vi "Example - DataType Datatype Check.vi"() -> ()   [LabVIEW 2017]
uses:
  API-String-Arugments-Support/API String Arguments Support.lvlib
panel:
  in  "String 32":string=" -4.86725 "
  out "error 16":errorcluster
  out "Data 15":cdb=-4.86725+0.0i
  out "String 31":string="-4.86725 +0i"
  in  "String 30":string="-3.14i "
  out "error 15":errorcluster
  out "Data 14":cdb=-3.14+0.0i
  out "String 29":string="-3.14 +0i"
  in  "String 28":string=" -4.86725 +3.14i "
  out "error 14":errorcluster
  out "Data 13":cdb=-4.86725+3.14i
  out "String 27":string="-4.86725 +3.14i"
  in  "String 26":string=" 4.86725 +3.14i "
  out "error 13":errorcluster
  out "Data 12":cdb=4.86725+3.14i
  out "String 25":string="4.86725 +3.14i"
  out "String 24":string="abcd"
  out "String 23":string="TRUE"
  out "String 22":string="66"
  out "String 21":string="3.1415926"
  out "String 20":string="bbbb"
  out "String 19":string="555 - ccccc"
  out "String 18":string="555 - ccccc"
  out "String 17":string="[3.12,4.11,5]"
  out "String 16":string="{Name:abc;Child.Name:ddd;Bool:FALSE}"
  out "String 15":string="C:\\ni-rt\\data\\a\\2023.07.25"
  out "String 14":string="[{Name:;Child.Name:ddd;Bool:FALSE},{Name:ddd;Child.Name:;Bool:TRUE}]"
  out "String 13":string="[3.12,4.113,2.3,5;3.12,5,2.3,0;3.12,4.11,5,0]"
  in  "String 12":string="[3.12,4.113,2.3,5;3.12,5,2.3;3.12,4.11,5]"
  out "error 12":errorcluster
  out "Data 11":dbl[][](array[numeric])=[[3.12, 4.113, 2.3, 5.0], [3.12, 5.0, 2.3, 0.0], [3.12, 4.11, 5.0, 0.0]]
  in  "String 11":string="[{Bool:Off;child.name:ddd},{Bool:On;name:ddd}]"
  out "error 11":errorcluster
  out "Data 10":T1(array[cluster])=[{"Name"="", "Child"={"Name"="ddd"}, "Bool"=FALSE}, {"Name"="ddd", "Child"={"Name"=""}, "Bool"=TRUE}]
  in  "String 10":string="C:\\ni-rt\\data\\a\\2023.07.25"
  out "error 10":errorcluster
  out "Data 9":path=path "C:/ni-rt/data/a/2023.07.25"
  in  "String 9":string="Bool:Off;child.name:ddd"
  out "error 9":errorcluster
  out "Data 8":T2={"Name"="abc", "Child"={"Name"="ddd"}, "Bool"=FALSE}
  in  "String 8":string="[3.12,4.11,5]"
  out "error 8":errorcluster
  out "Data 4":dbl[](array[numeric])=[3.12, 4.11, 5.0]
  in  "String 7":string="ccccc"
  out "error 7":errorcluster
  out "Data 7":enum16{"1 - aaaa", "2 - bbbb", "555 - ccccc"}(ring)=enum."555 - ccccc"
  in  "String 6":string="555"
  out "error 6":errorcluster
  out "Data 6":enum16{"1 - aaaa", "2 - bbbb", "555 - ccccc"}(ring)=enum."555 - ccccc"
  in  "String 5":string="bbbb"
  out "error 5":errorcluster
  out "Data 5":enum16{"aaaa", "bbbb", "ccccc"}(ring)=enum."bbbb"
  in  "String 4":string="3.1415926"
  out "error 4":errorcluster
  out "Data 4":dbl=3.1415926
  in  "String 3":string="0x42"
  out "error 3":errorcluster
  out "Data 3":i32=66
  in  "String 2":string="Enable"
  out "error 2":errorcluster
  out "Data 2":bool=TRUE
  out "Data 1":string="abcd"
  out "error 1":errorcluster
  in  "String":string="abcd"
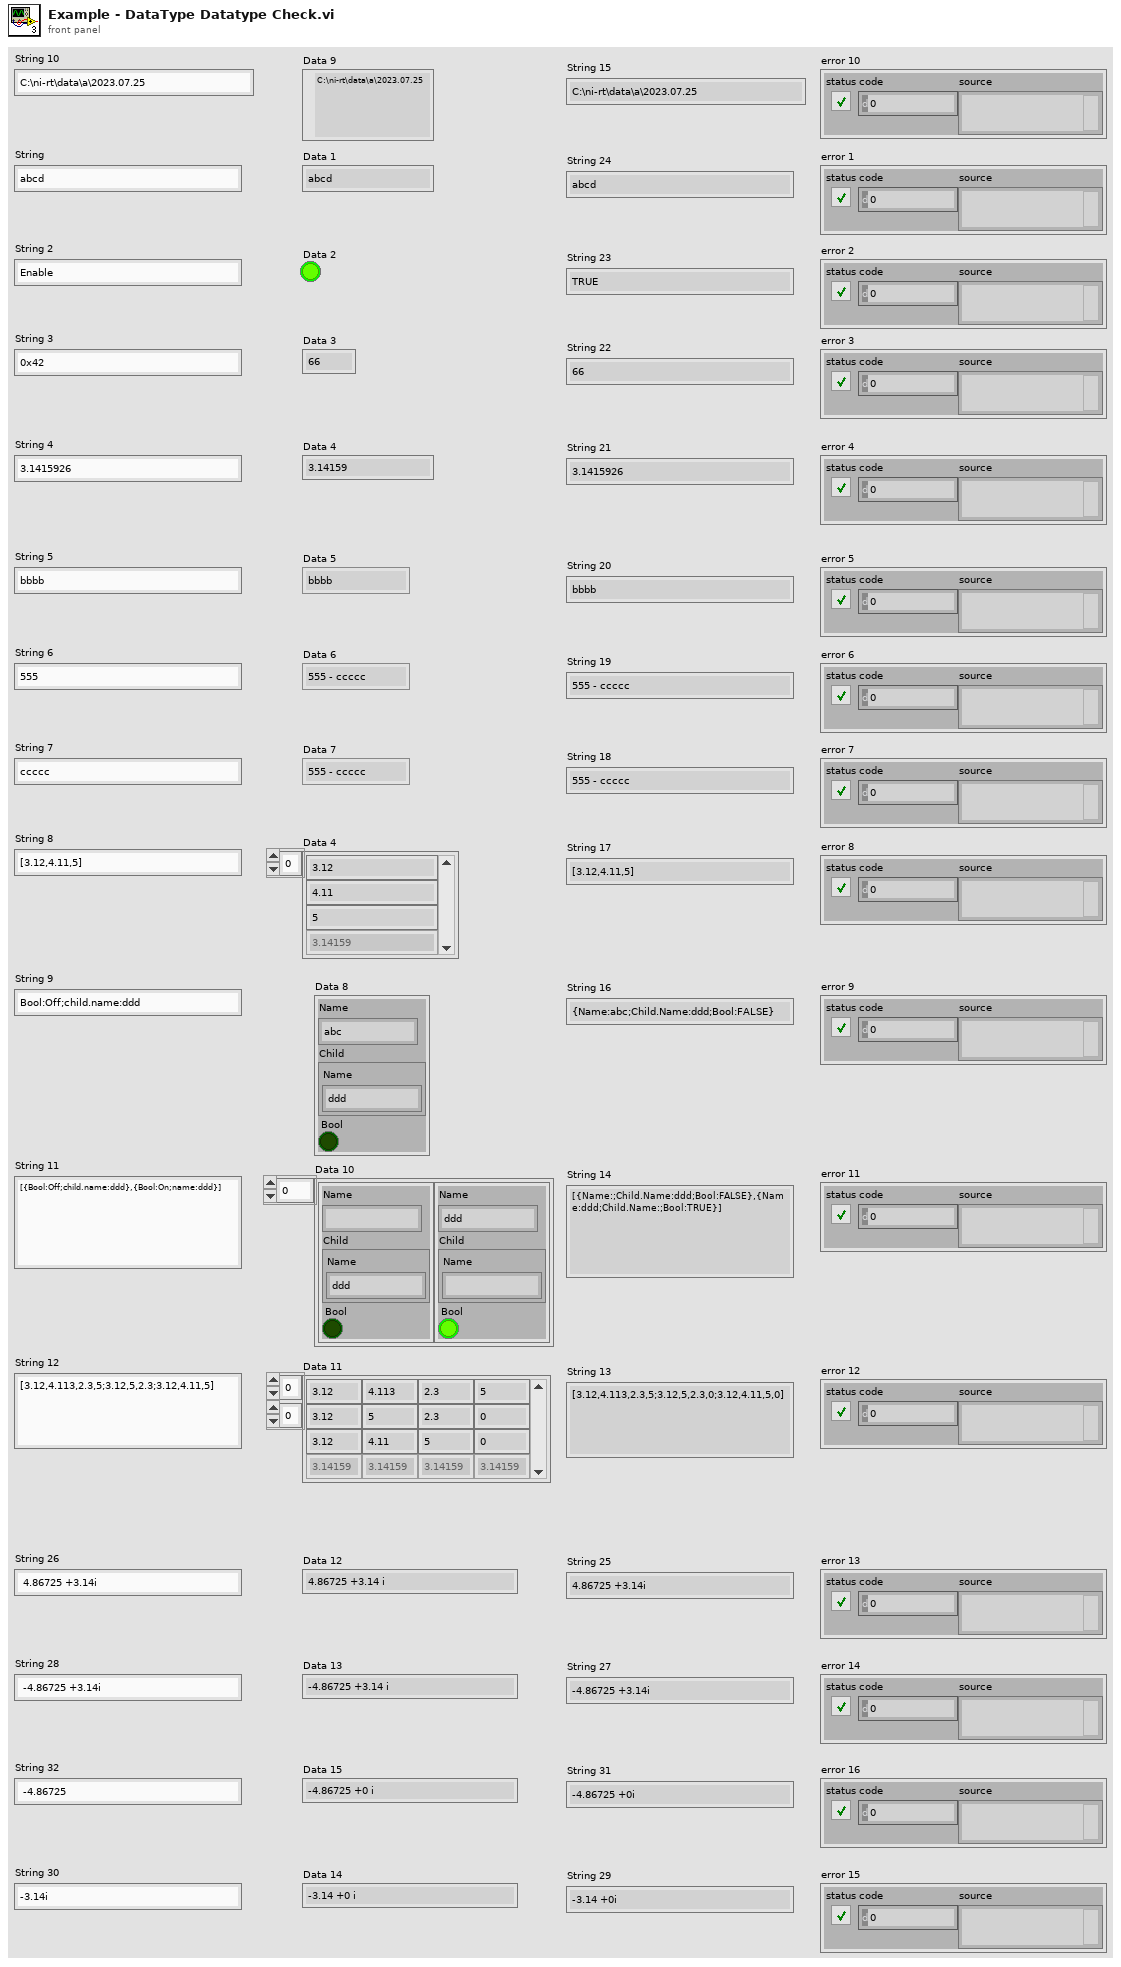
[diagram p1: front panel]
types:
  T1 = cluster{"Name":string, "Child":cluster{"Name":string}, "Bool":bool}[]
  T2 = cluster{"Name":string, "Child":cluster{"Name":string}, "Bool":bool}
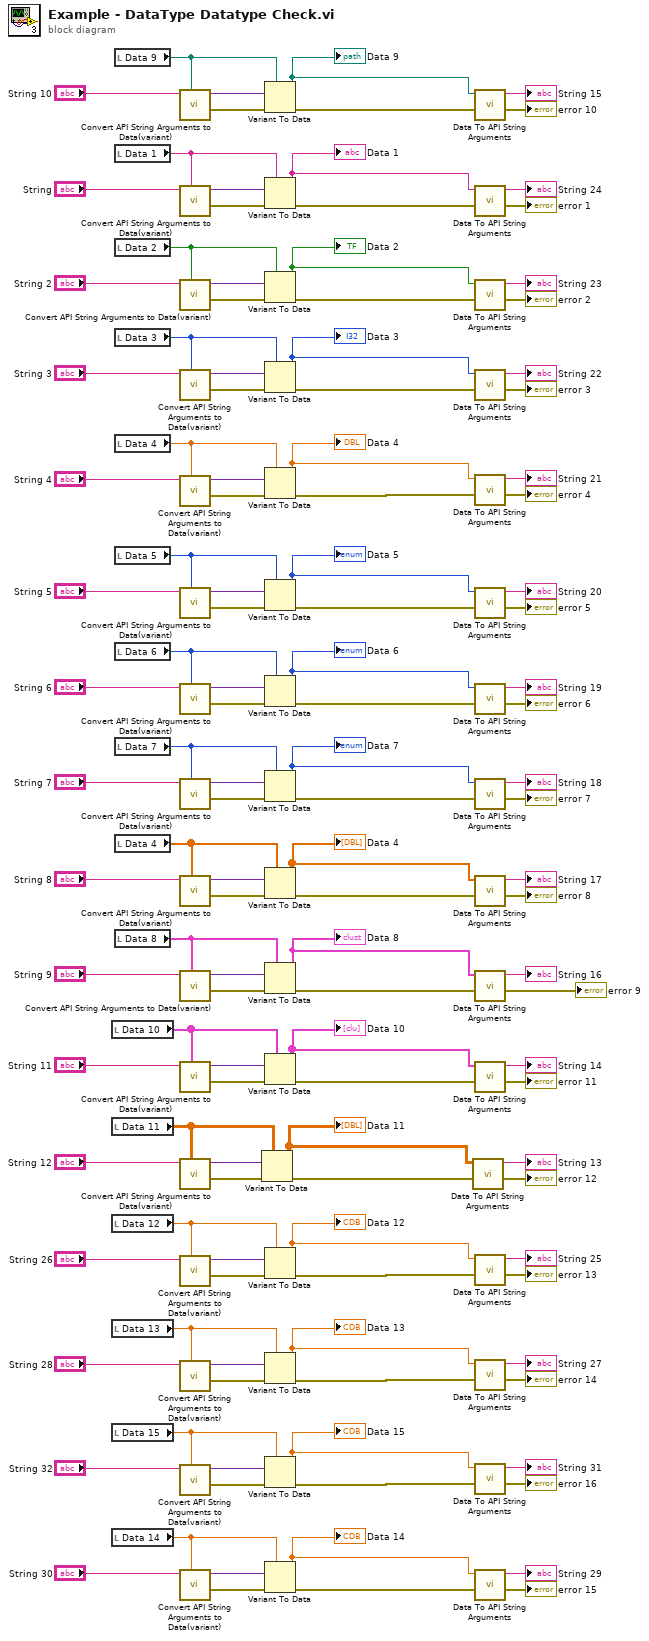
[diagram p0: block diagram]
diagram:
  n1 = local read "Data 10"() -> (w85:T1)
  n2 = local read "Data 11"() -> (w81:dbl[][])
  n3 = local read "Data 12"() -> (w25:cdb)
  n4 = local read "Data 13"() -> (w24:cdb)
  n5 = local read "Data 15"() -> (w8:cdb)
  n6 = local read "Data 14"() -> (w9:cdb)
  n7 = local read "Data 9"() -> (w89:path)
  n8 = local read "Data 1"() -> (w128:string)
  n9 = local read "Data 2"() -> (w127:bool)
  n10 = local read "Data 3"() -> (w126:i32)
  n11 = local read "Data 4"() -> (w125:dbl)
  n12 = local read "Data 5"() -> (w124:enum16{"aaaa", "bbbb", "ccccc"})
  n13 = local read "Data 6"() -> (w123:enum16{"1 - aaaa", "2 - bbbb", "555 - ccccc"})
  n14 = local read "Data 7"() -> (w122:enum16{"1 - aaaa", "2 - bbbb", "555 - ccccc"})
  n15 = local read "Data 4"() -> (w121:dbl[])
  n16 = local read "Data 8"() -> (w120:T2)
  n17 = call "Convert API String Arguments to Data(variant).vi"("Type"=w89, "String"="String 10") -> ("error"=w91:errorcluster, "Data"=w90:variant)  [unwired: 8 in]
  n18 = call "Convert API String Arguments to Data(variant).vi"("Type"=w128, "String"="String") -> ("error"=w94:errorcluster, "Data"=w95:variant)  [unwired: 8 in]
  n19 = call "Convert API String Arguments to Data(variant).vi"("Type"=w127, "String"="String 2") -> ("error"=w118:errorcluster, "Data"=w117:variant)  [unwired: 8 in]
  n20 = call "Convert API String Arguments to Data(variant).vi"("Type"=w126, "String"="String 3") -> ("error"=w115:errorcluster, "Data"=w116:variant)  [unwired: 8 in]
  n21 = call "Convert API String Arguments to Data(variant).vi"("Type"=w125, "String"="String 4") -> ("error"=w113:errorcluster, "Data"=w114:variant)  [unwired: 8 in]
  n22 = call "Convert API String Arguments to Data(variant).vi"("Type"=w124, "String"="String 5") -> ("error"=w111:errorcluster, "Data"=w112:variant)  [unwired: 8 in]
  n23 = call "Convert API String Arguments to Data(variant).vi"("Type"=w123, "String"="String 6") -> ("error"=w109:errorcluster, "Data"=w110:variant)  [unwired: 8 in]
  n24 = call "Convert API String Arguments to Data(variant).vi"("Type"=w122, "String"="String 7") -> ("error"=w107:errorcluster, "Data"=w108:variant)  [unwired: 8 in]
  n25 = call "Convert API String Arguments to Data(variant).vi"("Type"=w121, "String"="String 8") -> ("error"=w105:errorcluster, "Data"=w106:variant)  [unwired: 8 in]
  n26 = call "Convert API String Arguments to Data(variant).vi"("Type"=w120, "String"="String 9") -> ("error"=w103:errorcluster, "Data"=w104:variant)  [unwired: 8 in]
  n27 = call "Convert API String Arguments to Data(variant).vi"("Type"=w85, "String"="String 11") -> ("error"=w87:errorcluster, "Data"=w86:variant)  [unwired: 8 in]
  n28 = call "Convert API String Arguments to Data(variant).vi"("Type"=w81, "String"="String 12") -> ("error"=w83:errorcluster, "Data"=w82:variant)  [unwired: 8 in]
  n29 = call "Convert API String Arguments to Data(variant).vi"("Type"=w25, "String"="String 26") -> ("error"=w27:errorcluster, "Data"=w26:variant)  [unwired: 8 in]
  n30 = call "Convert API String Arguments to Data(variant).vi"("Type"=w24, "String"="String 28") -> ("error"=w22:errorcluster, "Data"=w23:variant)  [unwired: 8 in]
  n31 = call "Convert API String Arguments to Data(variant).vi"("Type"=w8, "String"="String 32") -> ("error"=w6:errorcluster, "Data"=w7:variant)  [unwired: 8 in]
  n32 = call "Convert API String Arguments to Data(variant).vi"("Type"=w9, "String"="String 30") -> ("error"=w11:errorcluster, "Data"=w10:variant)  [unwired: 8 in]
  n33 = Variant To Data(error in=w83, type=w81, Variant=w82) -> (data=w41:dbl[][], error out=w45:errorcluster)
  "Data 11" <- w41
  n34 = Variant To Data(error in=w91, type=w89, Variant=w90) -> (data=w33:path, error out=w56:errorcluster)
  "Data 9" <- w33
  n35 = Variant To Data(error in=w94, type=w128, Variant=w95) -> (data=w34:string, error out=w55:errorcluster)
  "Data 1" <- w34
  n36 = Variant To Data(error in=w118, type=w127, Variant=w117) -> (data=w35:bool, error out=w54:errorcluster)
  "Data 2" <- w35
  n37 = Variant To Data(error in=w115, type=w126, Variant=w116) -> (data=w36:i32, error out=w53:errorcluster)
  "Data 3" <- w36
  n38 = Variant To Data(error in=w113, type=w125, Variant=w114) -> (data=w37:dbl, error out=w52:errorcluster)
  "Data 4" <- w37
  n39 = Variant To Data(error in=w111, type=w124, Variant=w112) -> (data=w40:enum16{"aaaa", "bbbb", "ccccc"}, error out=w51:errorcluster)
  "Data 5" <- w40
  n40 = Variant To Data(error in=w109, type=w123, Variant=w110) -> (data=w39:enum16{"1 - aaaa", "2 - bbbb", "555 - ccccc"}, error out=w50:errorcluster)
  "Data 6" <- w39
  n41 = Variant To Data(error in=w107, type=w122, Variant=w108) -> (data=w38:enum16{"1 - aaaa", "2 - bbbb", "555 - ccccc"}, error out=w49:errorcluster)
  "Data 7" <- w38
  n42 = Variant To Data(error in=w105, type=w121, Variant=w106) -> (data=w44:dbl[], error out=w48:errorcluster)
  "Data 4" <- w44
  n43 = Variant To Data(error in=w103, type=w120, Variant=w104) -> (data=w43:T2, error out=w47:errorcluster)
  "Data 8" <- w43
  n44 = Variant To Data(error in=w87, type=w85, Variant=w86) -> (data=w42:T1, error out=w46:errorcluster)
  "Data 10" <- w42
  n45 = Variant To Data(error in=w27, type=w25, Variant=w26) -> (data=w32:cdb, error out=w31:errorcluster)
  "Data 12" <- w32
  n46 = Variant To Data(error in=w22, type=w24, Variant=w23) -> (data=w17:cdb, error out=w18:errorcluster)
  "Data 13" <- w17
  n47 = Variant To Data(error in=w6, type=w8, Variant=w7) -> (data=w1:cdb, error out=w2:errorcluster)
  "Data 15" <- w1
  n48 = Variant To Data(error in=w11, type=w9, Variant=w10) -> (data=w16:cdb, error out=w15:errorcluster)
  "Data 14" <- w16
  n49 = call "Data To API String Arguments.vi"("error in (no error)"=w45, "data"=w41) -> ("error out"=→"error 12":errorcluster, "String"=→"String 13":string)  [unwired: 8 in]
  n50 = call "Data To API String Arguments.vi"("error in (no error)"=w56, "data"=w33) -> ("error out"=→"error 10":errorcluster, "String"=→"String 15":string)  [unwired: 8 in]
  n51 = call "Data To API String Arguments.vi"("error in (no error)"=w55, "data"=w34) -> ("error out"=→"error 1":errorcluster, "String"=→"String 24":string)  [unwired: 8 in]
  n52 = call "Data To API String Arguments.vi"("error in (no error)"=w54, "data"=w35) -> ("error out"=→"error 2":errorcluster, "String"=→"String 23":string)  [unwired: 8 in]
  n53 = call "Data To API String Arguments.vi"("error in (no error)"=w53, "data"=w36) -> ("error out"=→"error 3":errorcluster, "String"=→"String 22":string)  [unwired: 8 in]
  n54 = call "Data To API String Arguments.vi"("error in (no error)"=w52, "data"=w37) -> ("error out"=→"error 4":errorcluster, "String"=→"String 21":string)  [unwired: 8 in]
  n55 = call "Data To API String Arguments.vi"("error in (no error)"=w51, "data"=w40) -> ("error out"=→"error 5":errorcluster, "String"=→"String 20":string)  [unwired: 8 in]
  n56 = call "Data To API String Arguments.vi"("error in (no error)"=w50, "data"=w39) -> ("error out"=→"error 6":errorcluster, "String"=→"String 19":string)  [unwired: 8 in]
  n57 = call "Data To API String Arguments.vi"("error in (no error)"=w49, "data"=w38) -> ("error out"=→"error 7":errorcluster, "String"=→"String 18":string)  [unwired: 8 in]
  n58 = call "Data To API String Arguments.vi"("error in (no error)"=w48, "data"=w44) -> ("error out"=→"error 8":errorcluster, "String"=→"String 17":string)  [unwired: 8 in]
  n59 = call "Data To API String Arguments.vi"("error in (no error)"=w47, "data"=w43) -> ("error out"=→"error 9":errorcluster, "String"=→"String 16":string)  [unwired: 8 in]
  n60 = call "Data To API String Arguments.vi"("error in (no error)"=w46, "data"=w42) -> ("error out"=→"error 11":errorcluster, "String"=→"String 14":string)  [unwired: 8 in]
  n61 = call "Data To API String Arguments.vi"("error in (no error)"=w31, "data"=w32) -> ("error out"=→"error 13":errorcluster, "String"=→"String 25":string)  [unwired: 8 in]
  n62 = call "Data To API String Arguments.vi"("error in (no error)"=w18, "data"=w17) -> ("error out"=→"error 14":errorcluster, "String"=→"String 27":string)  [unwired: 8 in]
  n63 = call "Data To API String Arguments.vi"("error in (no error)"=w2, "data"=w1) -> ("error out"=→"error 16":errorcluster, "String"=→"String 31":string)  [unwired: 8 in]
  n64 = call "Data To API String Arguments.vi"("error in (no error)"=w15, "data"=w16) -> ("error out"=→"error 15":errorcluster, "String"=→"String 29":string)  [unwired: 8 in]
